vi "Generate Average Coverage String.vi"(8 "error in (no error)":errorcluster, 11 "Coverage Analyzer Result View in":refnum<class "Coverage Analyzer Result View.lvclass">) -> (0 "error out":errorcluster, 2 "Fraction of VIs Executed":string, 3 "Coverage Analyzer Result View out":refnum<class "Coverage Analyzer Result View.lvclass">)   [LabVIEW 2020, in "Coverage Analyzer.lvlib" / "Coverage Analyzer Result View.lvclass"]
uses:
  Coverage Analyzer Result View.lvclass
  Coverage Analyzer Result View.lvclass/Coverage Analyzer Result View.ctl
  <vilib>/Analysis/baseanly.llb/Mean (DBL).vi
  <vilib>/Analysis/NI_AALBase.lvlib
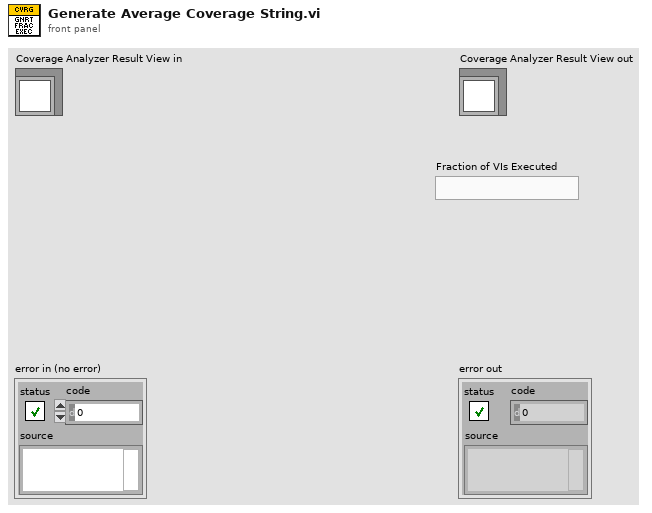
[diagram p1: front panel]
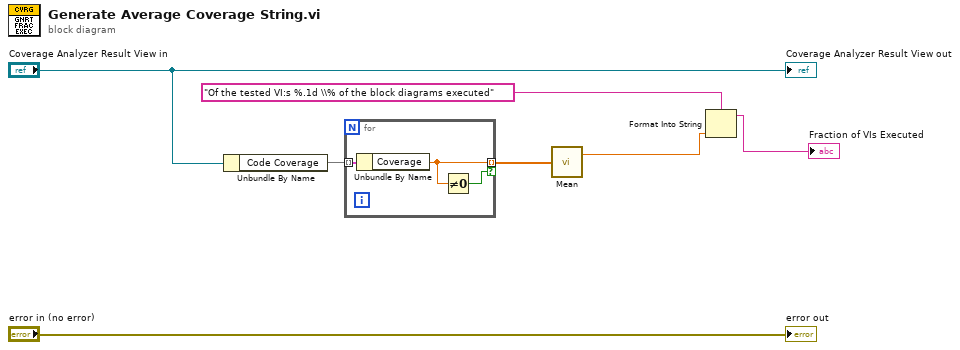
[diagram p0: block diagram]
diagram:
  n1 = Unbundle By Name("Coverage Analyzer Result View in") -> ("Code Coverage"=w3:map{path, dbl})
  n2 = for {
    tunnel: w3 -> [w10] mode=indexing
    tunnel: [w9] -> w2 mode=indexing if=w8
    n3 = Unbundle By Name(w10) -> ("Coverage"=w9:dbl)
    n4 = Not Equal To 0?(x=w9) -> (x != 0?=w8:bool)
  }
  n5 = call-poly <vilib>:"Mean.vi"("X"=w2) -> ("mean"=w1:dbl)  [unwired: 1 out]
  n6 = Format Into String(format string="Of the tested VI:s %.1d \\% of the block diagrams executed", w1) -> (resulting string=→"Fraction of VIs Executed":string)  [unwired: 2 in, 1 out]
  "error out" <- "error in (no error)"
  "Coverage Analyzer Result View out" <- "Coverage Analyzer Result View in"
